vi "From CSV File.vi"(8 "error in (no error)":errorcluster, 9 "Path":path, 10 "engine configuration":refnum<class "engine configuration.lvclass">, 11 "DAQmx Module Editor Node in":refnum<class "DAQmx Module editor node.lvclass">) -> (0 "error out":errorcluster, 1 "Update":bool, 2 "engine out":refnum<class "engine configuration.lvclass">, 3 "DAQmx Module Editor Node out":refnum<class "DAQmx Module editor node.lvclass">)   [LabVIEW 2015, in "DAQmx Module editor node.lvclass"]
uses:
  DAQmx Module editor node.lvclass
  <vilib>/NI/Module Execution Interface/Engine Configuration/engine configuration.lvclass
  module/configuration/Daqmx Module configuration.lvclass
  <vilib>/NI/Configuration Framework/serializable configuration/NISE_CEF_serializable configuration.lvclass/NISE_CEF_serializable configuration.ctl
  module/configuration/Daqmx Module configuration.lvclass/Daqmx Module configuration.ctl
  <vilib>/NI/Tag Bus/tag/tag descriptor.lvclass/tag descriptor.ctl
  <vilib>/Utility/LVClass/Get LV Class Name.vi
  <vilib>/NI/Configuration Framework/error generator/NISE_error generator.vi
  <vilib>/NI/Tag Bus Module Framework/channel/TBM channel.lvclass
  <vilib>/NI/Configuration Framework/serializable configuration/NISE_CEF_serializable configuration.lvclass
  <vilib>/NI/Tag Bus/tag/tag descriptor.lvclass
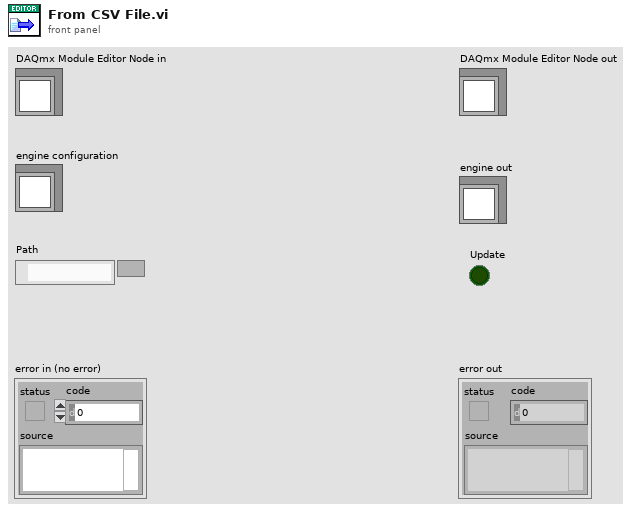
[diagram p1: front panel]
types:
  T1 = typedef "DAQmx Module Configuration.lvclass/Line.ctl" = cluster{"Channel Array":refnum<class "TBM channel.lvclass">[], "Physical Channel":string, "Measurement Type":T2, "Parameters":T3}
  T2 = typedef "DAQmx Module Configuration.lvclass/Measurement Type.ctl" = enum16{"Digital Input", "Digital Output", "Voltage Input", "Voltage Output", "Current Input", "Current Output", "RTD", "Thermocouple", "Strain", "PWM"}
  T3 = typedef "DAQmx Module Configuration.lvclass/Parameters.ctl" = cluster{"Digital Config":cluster{"Invert Lines?":bool}, "Voltage Config":cluster{"Maximum Value (V)":dbl, "Minimum Value (V)":dbl, "in terminal configuration (V)":i32, "out terminal configuration (V)":i32}, "Current Config":cluster{"Maximum Value (A)":dbl, "Minimum Value (A)":dbl, "shunt resistor location":i32, "input terminal configuration (C)":i32, "external shunt resistor value":dbl}, "RTD Config":cluster{"Maximum Value (°C)":dbl, "Minimum Value (°C)":dbl, "resistance configuration":i32, "r0":dbl, "current excitation value":dbl, "rtd type":i32, "current excitation source":i32}, "Thermocouple Config":cluster{"Minimum Value (C)":dbl, "Maximum Value (C)":dbl, "thermocouple type":i32, "cjc source":i32, "cjc value":dbl}, "Strain Config":cluster{"Maximum Value":dbl, "Minimum Value":dbl, "bridge information":cluster{"strain configuration":i32, "lead wire resistance":dbl, "initial bridge voltage":dbl, "voltage excitation source":i32, "voltage excitation value":dbl}, "strain gage information":cluster{"gage factor":dbl, "nominal gage resistance":dbl, "poisson ratio":dbl}}, "PWM Config":cluster{"Idle State":bool}}
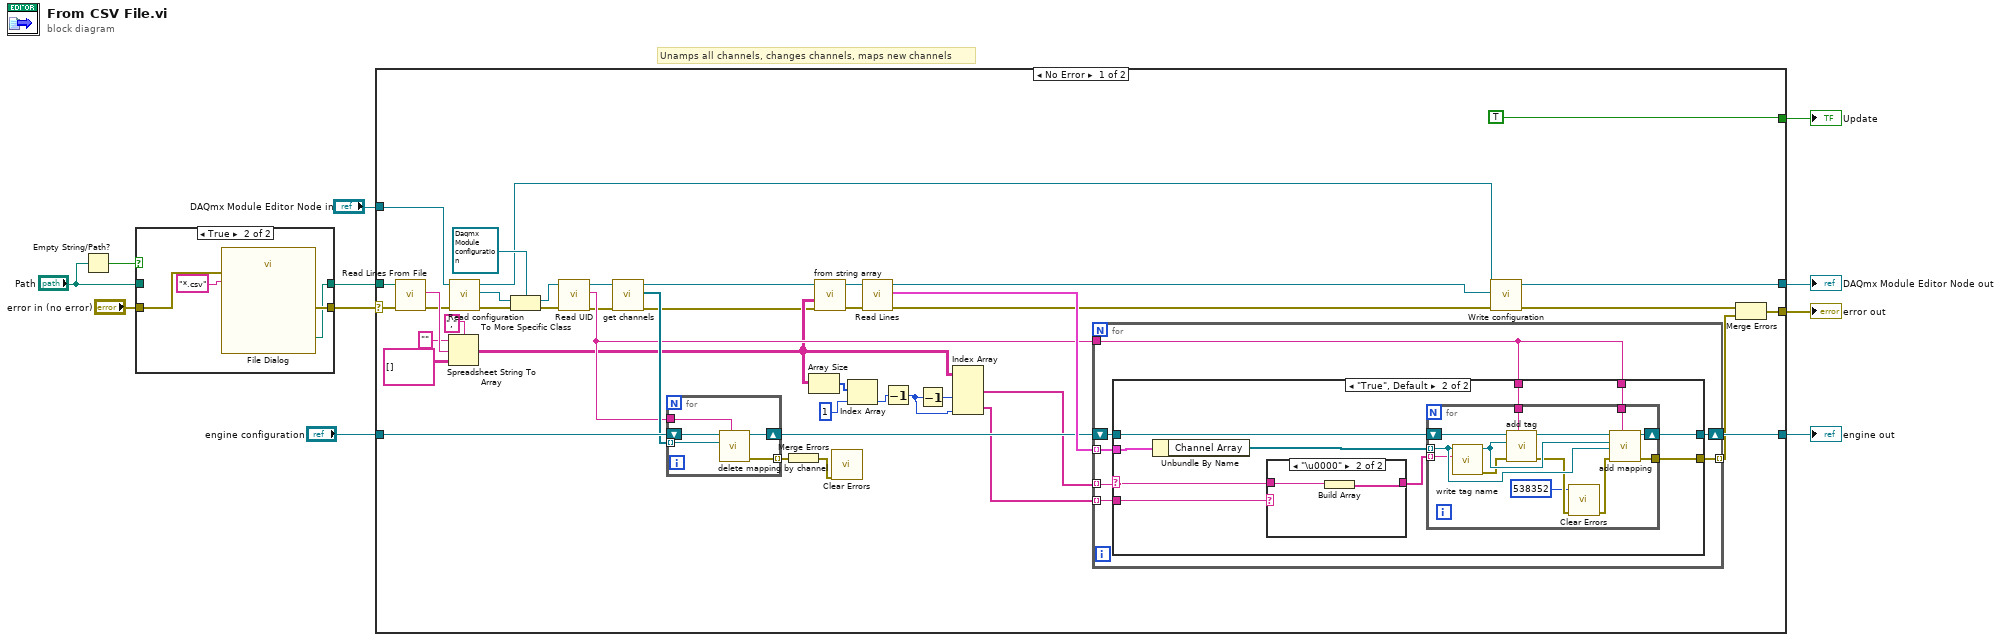
[diagram p0: block diagram]
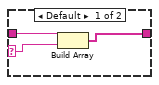
[diagram p4: hidden frame]
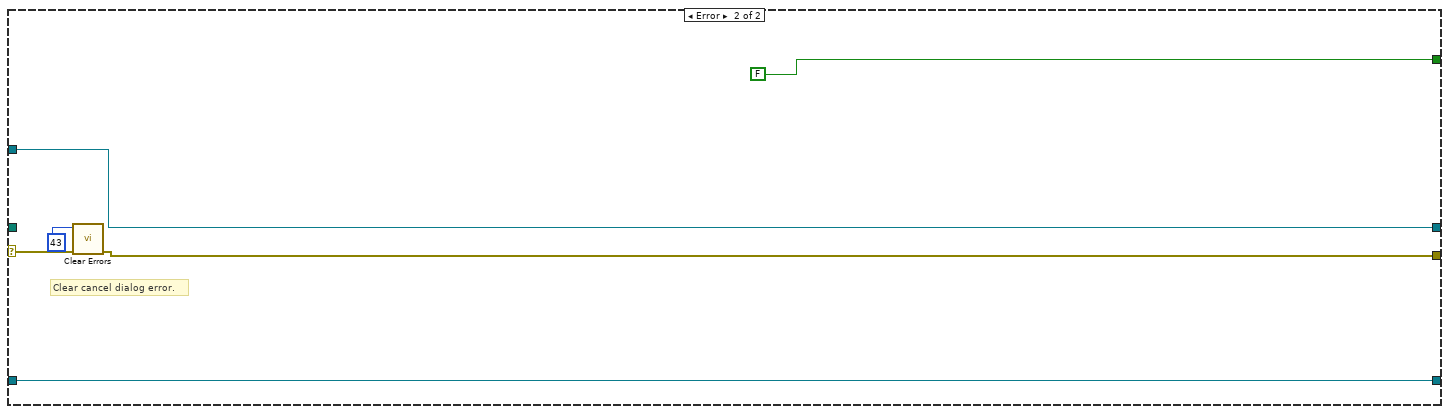
[diagram p5: hidden frame]
diagram:
  # "Unamps all channels, changes channels, maps new channels"
  n1 = Empty String/Path?(string/path="Path") -> (empty?=w11:bool)
  n2 = case shown="True" w11 {
    tunnel: "error in (no error)" -> [w12 w16]
    tunnel: [w12 w15] -> w10
    tunnel: [w13 w14] -> w9
    tunnel: "Path" -> [w13 _]
    frame False {
    }
    frame True {
      n3 = call "File Dialog"("error in"=w16, "pattern (all files)"="*.csv") -> ("selected path"=w14:path, "error out"=w15:errorcluster)  [unwired: 10 in, 2 out]
    }
  }
  n4 = case shown="No Error" w10 {
    selector: w10 -> [w53 w104]
    tunnel: [w38 w103] -> w4
    tunnel: [w25 w106] -> w6
    tunnel: "DAQmx Module Editor Node in" -> [w32 w106]
    tunnel: w9 -> [w58 _]
    tunnel: [TRUE ("Update") FALSE ("Update")] -> w5
    tunnel: "engine configuration" -> [w50 w101]
    tunnel: [w41 w101] -> w1
    frame No Error {
      n5 = call <vilib>:"Read Lines From File.vi"("file path (dialog if empty)"=w58, "error in (not an error)"=w53) -> ("line string"=w56:string, "error out"=w31:errorcluster)  [unwired: 5 in, 1 out]
      n6 = Spreadsheet String To Array(delimiter (Tab)=",", format string="", spreadsheet string=w56, array type (2D Dbl)=string[][] [] ("type (empty)")) -> (array=w36:string[][])
      n7 = call-dynamic "Read configuration.vi"("error in"=w31, "Daqmx Module editor node in"=w32) -> ("error out"=w29:errorcluster, "configuration"=w30:refnum<class "NISE_CEF_serializable configuration.lvclass">, "Daqmx Module editor node out"=w28:refnum<class "DAQmx Module editor node.lvclass">)  [unwired: 7 in]
      n8 = To More Specific Class(target class=refnum<class "Daqmx Module configuration.lvclass"> refnum ("Daqmx Module configuration"), reference=w30, error in=w29) -> (specific class reference=w52:refnum<class "Daqmx Module configuration.lvclass">, error out=w46:errorcluster)
      n9 = call <vilib>:"Read UID.vi"("error in"=w46, "configuration in"=w52) -> ("error out"=w22:errorcluster, "instance id"=w39:string, "configuration out"=w51:refnum<class "Daqmx Module configuration.lvclass">)  [unwired: 7 in]
      n10 = call-dynamic "get channels.vi"("Daqmx Module configuration in"=w51) -> ("channels"=w49:refnum<class "TBM channel.lvclass">[], "Daqmx Module configuration out"=w47:refnum<class "Daqmx Module configuration.lvclass">)  [unwired: 9 in]
      n11 = for {
        tunnel: w39 -> [w99]
        tunnel: w49 -> [w98] mode=indexing
        tunnel: [w97] -> w48 mode=indexing
        shift-right: [w96] -> w42
        shift-left: w50 -> [w100]
        n12 = call <vilib>:"delete mapping by channel.vi"("owner ID"=w99, "channel"=w98, "engine configuration in"=w100) -> ("error out"=w97:errorcluster, "engine configuration out"=w96:refnum<class "engine configuration.lvclass">)  [unwired: 7 in]
      }
      n13 = Merge Errors(w48) -> (w23:errorcluster)
      n14 = Array Size(array=w36) -> (size(s)=w35:i32[])
      n15 = call-dynamic "from string array.vi"("error in (no error)"=w22, "String Array"=w36, "module configuration in"=w47) -> ("error out"=w40:errorcluster, "module configuration out"=w45:refnum<class "Daqmx Module configuration.lvclass">)  [unwired: 7 in]
      n16 = call <vilib>:"Clear Errors.vi"("error in (no error)"=w23) -> ()  [unwired: 5 in, 2 out]
      n17 = Index Array(array=w35, index=1) -> (element=w33:i32)
      n18 = call "Read Lines.vi"("error in (no error)"=w40, "Daqmx Module configuration in"=w45) -> ("error out"=w26:errorcluster, "Lines"=w43:T1[], "Daqmx Module configuration out"=w27:refnum<class "Daqmx Module configuration.lvclass">)  [unwired: 7 in]
      n19 = Decrement(x=w33) -> (x-1=w20:i32)
      n20 = Decrement(x=w20) -> (x-1=w21:i32)
      n21 = Index Array(array=w36, index (col) #1=w21, index (col) #2=w20) -> (element #1=w19:string[], element #2=w18:string[])  [unwired: 2 in]
      n22 = for {
        tunnel: w43 -> [w66] mode=indexing
        tunnel: w19 -> [w62] mode=indexing
        shift-right: [w65] -> w41
        shift-left: w42 -> [w63]
        tunnel: w39 -> [w61]
        tunnel: [w64] -> w37 mode=indexing
        tunnel: w18 -> [w60] mode=indexing
        n23 = case shown="\"True\", Default" w62 {
          selector: w62 -> [_ w70]
          tunnel: w66 -> [_ w77]
          tunnel: [w67 w76] -> w65
          tunnel: w61 -> [_ w75]
          tunnel: [_ w74] -> w64
          tunnel: w63 -> [w67 w73]
          tunnel: w61 -> [_ w71]
          tunnel: w60 -> [_ w68]
          frame "" {
          }
          frame "True", Default {
            n24 = Unbundle By Name(w77) -> ("Channel Array"=w72:refnum<class "TBM channel.lvclass">[])
            n25 = case shown="\"\"" w68 {
              selector: w68 -> [w79 _]
              tunnel: w70 -> [w80 w82]
              tunnel: [w78 w81] -> w69
              frame Default {
                n26 = Build Array(w80, w79) -> (w78:string[])
              }
              frame "\u0000" {
                n27 = Build Array(w82) -> (w81:string[])
              }
            }
            n28 = for {
              tunnel: w75 -> [w94]
              tunnel: [w93] -> w74
              tunnel: w72 -> [w89] mode=indexing
              tunnel: w69 -> [w84] mode=indexing
              shift-right: [w95] -> w76
              shift-left: w73 -> [w92]
              tunnel: w71 -> [w83]
              n29 = call <vilib>:"write tag name.vi"("name"=w84, "system tag in"=w89) -> ("error out"=w88:errorcluster, "system tag out"=w90:refnum<class "TBM channel.lvclass">)  [unwired: 8 in]
              n30 = call-dynamic "add tag.vi"("owner ID"=w83, "error in"=w88, "tag descriptor"=w90, "engine configuration in"=w92) -> ("error out"=w87:errorcluster, "engine configuration out"=w91:refnum<class "engine configuration.lvclass">)  [unwired: 6 in]
              n31 = call <vilib>:"Clear Errors.vi"("error in (no error)"=w87, "specific error code to clear (0: all)"=538352) -> ("error out"=w86:errorcluster)  [unwired: 4 in, 1 out]
              n32 = call-dynamic "add mapping.vi"("owner ID"=w94, "error in"=w86, "channel"=w89, "tag descriptor"=w90, "engine configuration"=w91) -> ("error out"=w93:errorcluster, "engine configuration out"=w95:refnum<class "engine configuration.lvclass">)  [unwired: 5 in]
            }
          }
        }
      }
      n33 = call-dynamic "Write configuration.vi"("error in"=w26, "configuration"=w27, "Daqmx Module editor node in"=w28) -> ("error out"=w24:errorcluster, "Daqmx Module editor node out"=w25:refnum<class "DAQmx Module editor node.lvclass">)  [unwired: 7 in]
      n34 = Merge Errors(w24, w37) -> (w38:errorcluster)
    }
    frame Error {
      # "Clear cancel dialog error."
      n35 = call <vilib>:"Clear Errors.vi"("error in (no error)"=w104, "specific error code to clear (0: all)"=43) -> ("error out"=w103:errorcluster)  [unwired: 4 in, 1 out]
    }
  }
  "error out" <- w4
  "DAQmx Module Editor Node out" <- w6
  "Update" <- w5
  "engine out" <- w1
